vi "Config.vi"(8 "error in (no error)":errorcluster, 9 "Conf. Gral.":T1, 10 "Array Parsed Expression":T3[](array[typedef]), 11 "Variable Data In":T2) -> (0 "error out":errorcluster, 1 "Conf. Gral. Out":T1, 2 "Array Parsed Expression Out":T3[](array[typedef]), 3 "Variable Data Out":T2)   [LabVIEW 2014, in "MathLoop.lvlib"]
doc: "Configura Auxiliares, mediciones, ctes y dimensiones."
uses:
  MathLoop.lvlib
  TypeDefs/ParsedExpression.ctl
  TypeDefs/typeMed.ctl
  TypeDefs/NumericData.ctl
  TypeDefs/Conf. Gral.ctl
panel:
  in  "Configuración General.":bool
  in  "Acept":bool
  in  "Cancelar":bool
  in  "Dimensiones de Patrón":bool
  in  "Constantes de Medición":bool
  in  "Medidas Auxiliares":bool
  in  "Definición de Mediciones M":bool
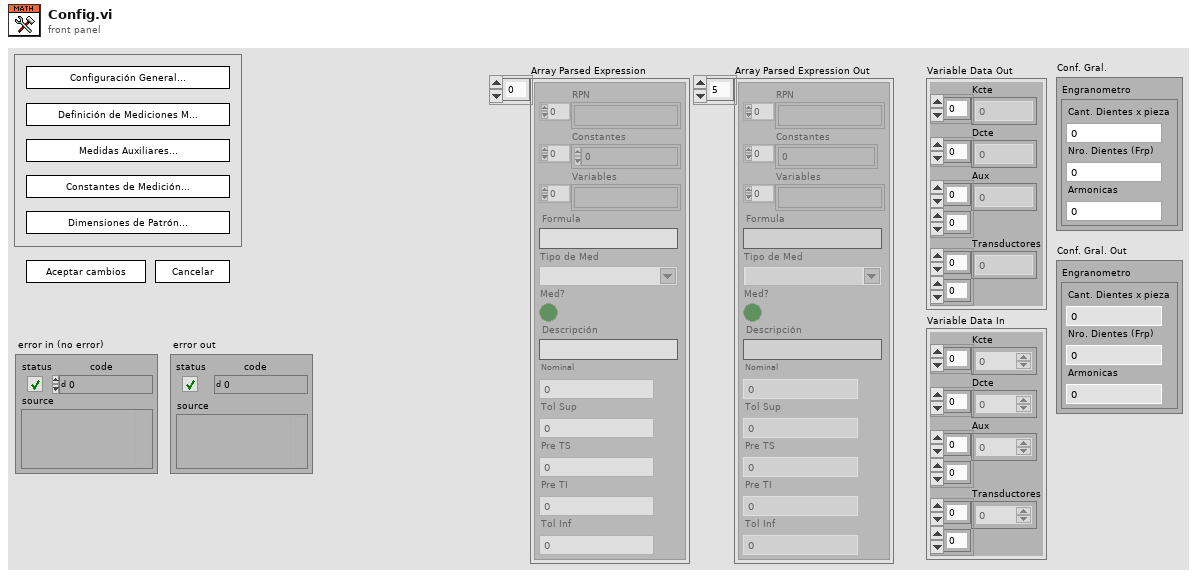
[diagram p1: front panel]
types:
  T1 = typedef "MathLoop.lvlib/Conf. Gral.ctl" = cluster{"Engranometro":cluster{"Cant. Dientes x pieza":i32, "Nro. Dientes (Frp)":i32, "Armonicas":i32}}
  T2 = typedef "MathLoop.lvlib/NumericData.ctl" = cluster{"Kcte":sgl[], "Dcte":sgl[], "Aux":sgl[][], "Transductores":sgl[][]}
  T3 = typedef "MathLoop.lvlib/ParsedExpression.ctl" = cluster{"RPN ":string[], "Constantes":sgl[], "Variables":string[], "Formula":string, "Tipo de Med":T4, "Med?":bool, "Descripción":string, "Nominal":sgl, "Tol Sup":sgl, "Pre TS":sgl, "Pre TI":sgl, "Tol Inf":sgl}
  T4 = typedef "MathLoop.lvlib/typeMed.ctl" = string
  T5 = cluster{"Kcte":sgl[], "Dcte":sgl[], "Aux":sgl[][], "Transductores":sgl[][]}
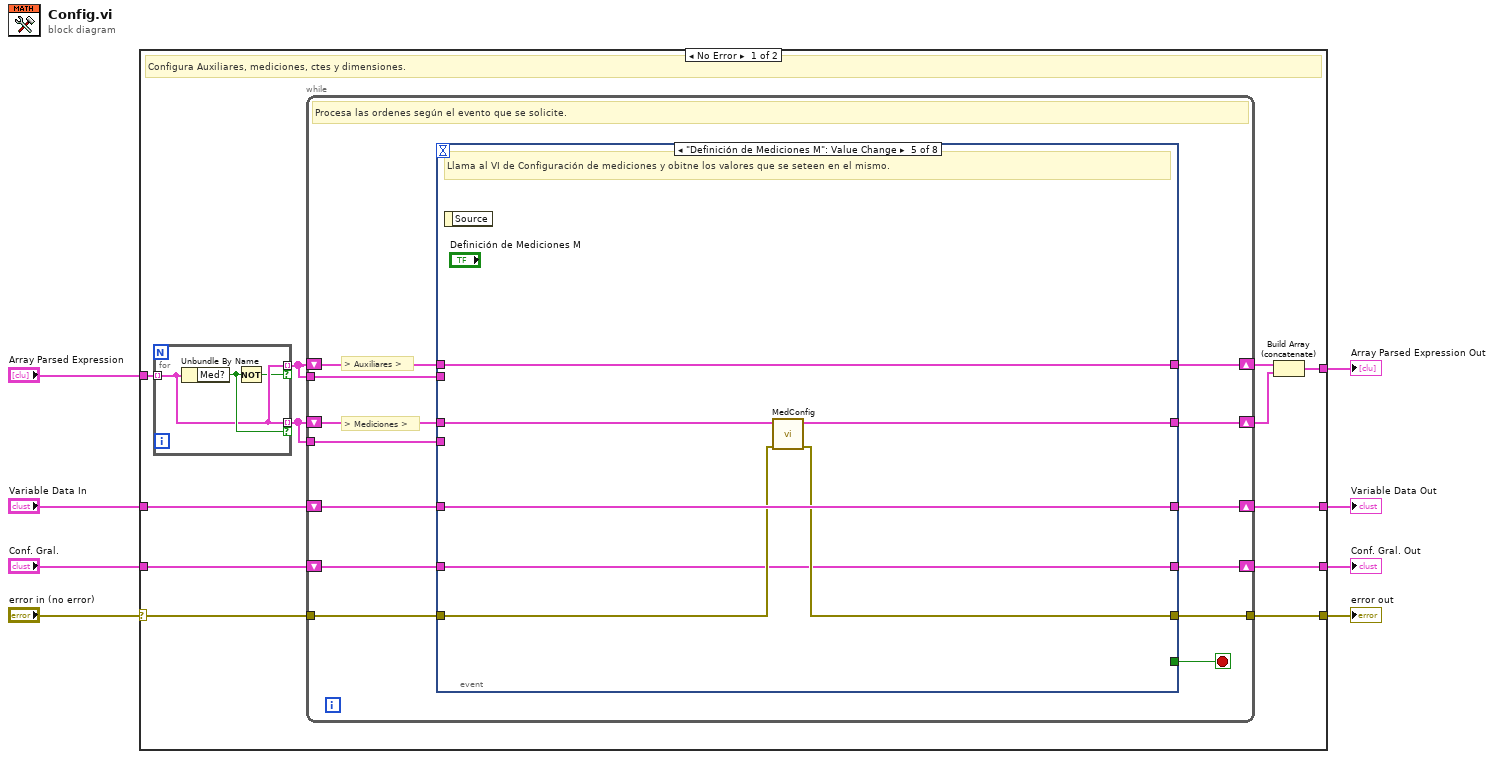
[diagram p0: block diagram]
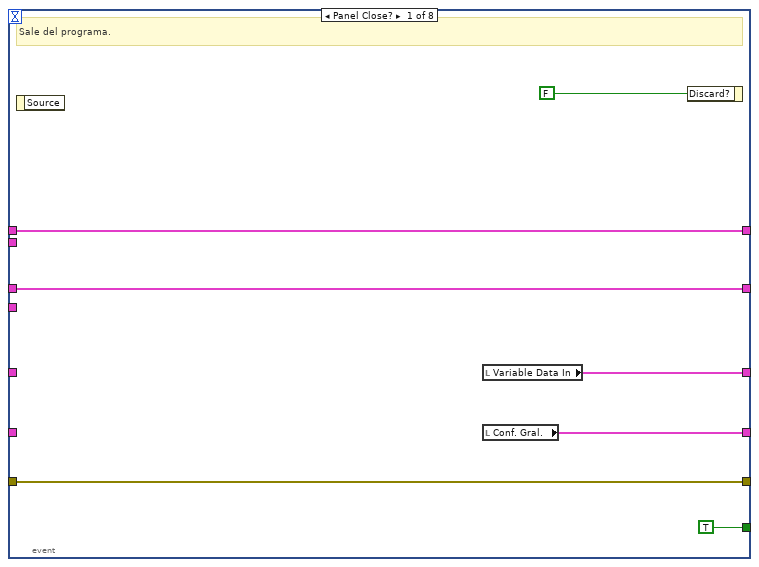
[diagram p2: hidden frame]
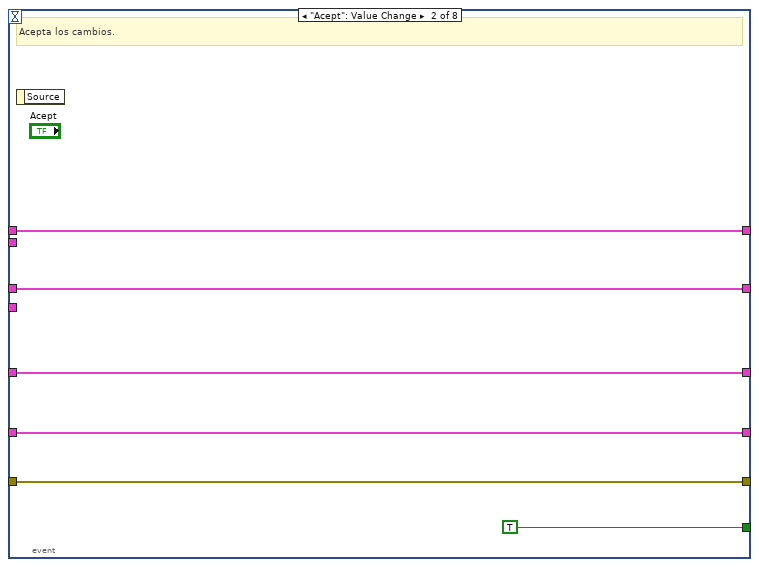
[diagram p3: hidden frame]
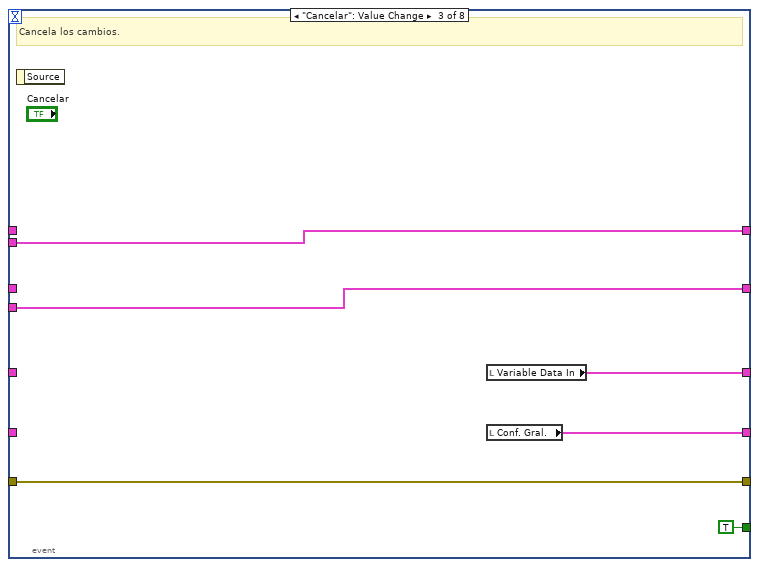
[diagram p4: hidden frame]
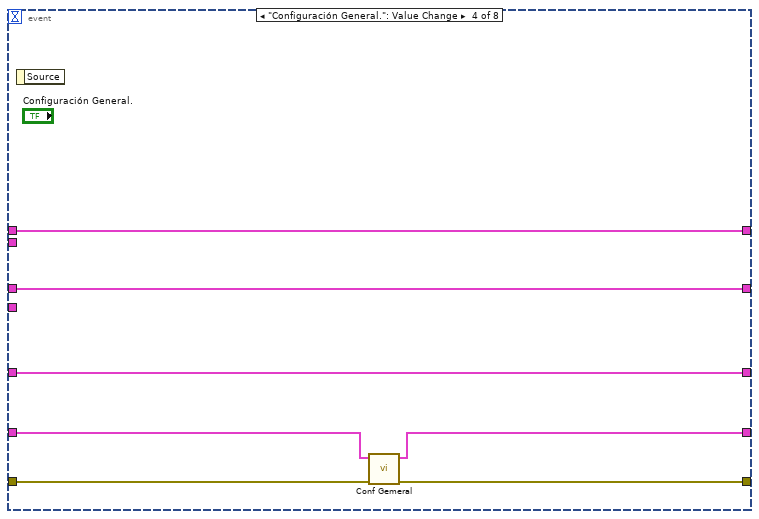
[diagram p5: hidden frame]
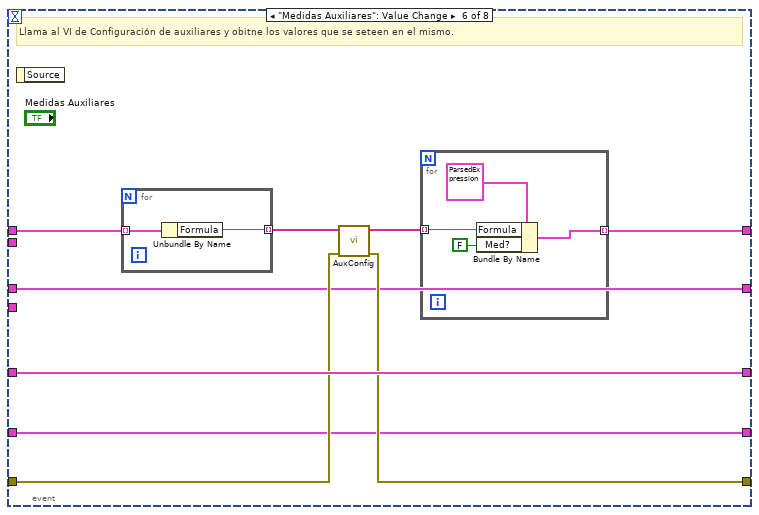
[diagram p6: hidden frame]
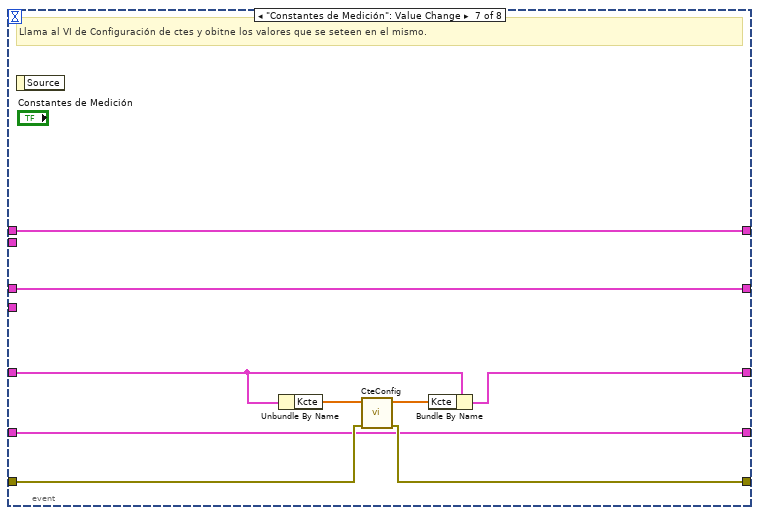
[diagram p7: hidden frame]
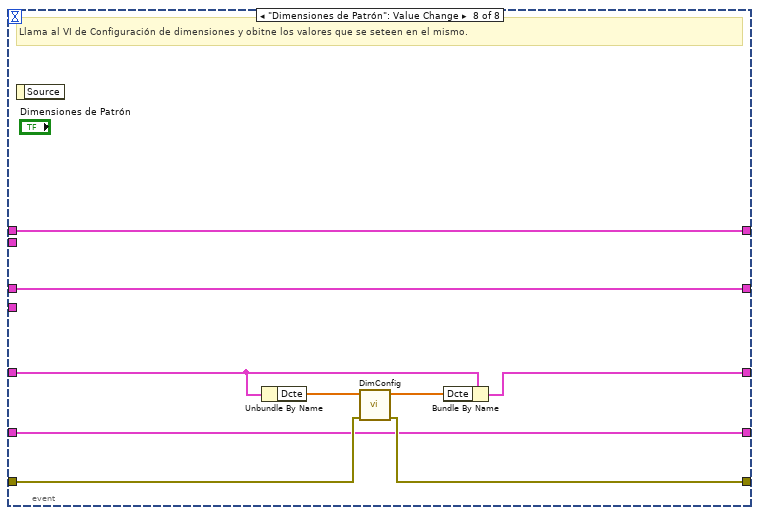
[diagram p8: hidden frame]
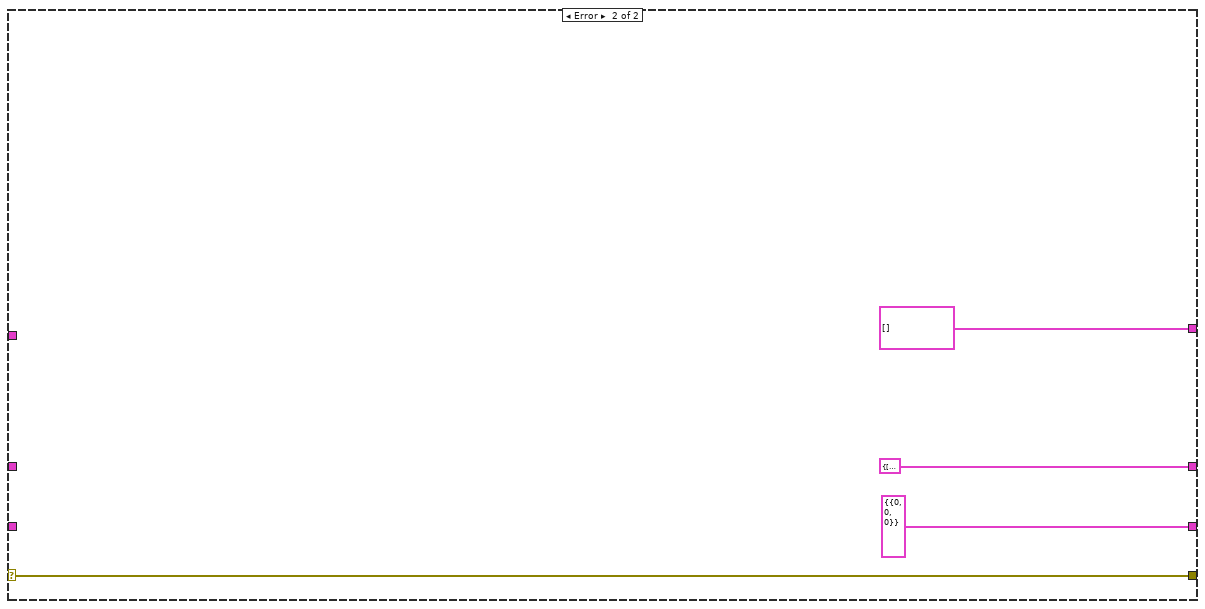
[diagram p9: hidden frame]
diagram:
  n1 = case shown="No Error" "error in (no error)" {
    selector: "error in (no error)" -> [w20 w106]
    tunnel: [w17 w106] -> w7
    tunnel: "Variable Data In" -> [w18 _]
    tunnel: "Array Parsed Expression" -> [w13 _]
    tunnel: [w19 T5 {"Kcte"=[], "Dcte"=[], "Aux"=[], "Transductores"=[]} ("Variable Data")] -> w3
    tunnel: [w14 T3[] [] ("Array Parsed Expression")] -> w5
    tunnel: [w10 T1 {"Engranometro"={"Cant. Dientes x pieza"=0, "Nro. Dientes (Frp)"=0, "Armonicas"=0}} ("Conf. Gral.")] -> w2
    tunnel: "Conf. Gral." -> [w9 _]
    frame No Error {
      # "Configura Auxiliares, mediciones, ctes y dimensiones."
      n2 = for {
        tunnel: w13 -> [w22] mode=indexing
        tunnel: [w22] -> w11 mode=indexing if=w23
        tunnel: [w22] -> w12 mode=indexing if=w21
        n3 = Unbundle By Name(w22) -> ("Med?"=w23:bool)
        n4 = Not(x=w23) -> (.not. x?=w21:bool)
      }
      n5 = while {
        tunnel: w20 -> [w36]
        tunnel: [w32] -> w17
        shift-right: [w33] -> w19
        shift-left: w18 -> [w34]
        shift-right: [w31] -> w16
        shift-left: w12 -> [w30]
        shift-right: [w29] -> w15
        shift-left: w11 -> [w28]
        tunnel: w12 -> [w27]
        tunnel: w11 -> [w26]
        shift-right: [w25] -> w10
        shift-left: w9 -> [w24]
        stop <- w35 stop-if-true
        # "> Mediciones >"
        # "> Auxiliares >"
        # "Procesa las ordenes según el evento que se solicite."
        n6 = event shown="[4] \"Definición de Mediciones M\": Value Change" {
          selector: _ -> [_ _ _ _ _ _ _ _]
          dyn-events: _ -> [_ _ _ _ _ _ _ _]
          timeout: _ -> [_ _ _ _ _ _ _ _]
          tunnel: [w42 w48 w55 w58 w66 w75 w90 w102] -> w32
          tunnel: w36 -> [w42 w48 w55 w59 w67 w76 w91 w101]
          tunnel: [TRUE ("Guardar") TRUE ("Guardar") TRUE ("Guardar") _ _ _ _ _] -> w35
          tunnel: w34 -> [_ w46 _ w62 w69 w78 w93 w100]
          tunnel: [w40 w46 w53 w62 w69 w78 w92 w99] -> w33
          tunnel: [w39 w47 w52 w61 w68 w72 w89 w98] -> w31
          tunnel: w30 -> [w39 w47 _ w61 w68 w71 w89 w98]
          tunnel: [w38 w45 w51 w60 w65 w74 w86 w95] -> w29
          tunnel: w28 -> [w38 w45 _ w60 w64 w74 w86 w95]
          tunnel: w27 -> [_ _ w52 _ _ _ _ _]
          tunnel: w26 -> [_ _ w51 _ _ _ _ _]
          tunnel: [w37 w44 w50 w57 w63 w70 w85 w94] -> w25
          tunnel: w24 -> [_ w44 _ w56 w63 w70 w85 w94]
          event Panel Close? {
            # "Sale del programa."
            n7 = event-data() -> ()  [unwired: 1 in, 1 out]
            n8 = local read "Variable Data In"() -> (w40:T2)
            n9 = local read "Conf. Gral."() -> (w37:T1)
            n10 = event-data("Discard?"=FALSE) -> ()  [unwired: 1 in, 1 out]
          }
          event "Acept": Value Change {
            # "Acepta los cambios."
            n11 = event-data() -> ()  [unwired: 1 in, 1 out]
          }
          event "Cancelar": Value Change {
            # "Cancela los cambios."
            n12 = event-data() -> ()  [unwired: 1 in, 1 out]
            n13 = local read "Variable Data In"() -> (w53:T2)
            n14 = local read "Conf. Gral."() -> (w50:T1)
          }
          event "Configuración General.": Value Change {
            n15 = event-data() -> ()  [unwired: 1 in, 1 out]
            n16 = call "Conf Gemeral.vi"("error in (no error)"=w59, "Conf. Gral."=w56) -> ("error out"=w58:errorcluster, "Conf. Gral. Out"=w57:T1)  [unwired: 8 in]
          }
          event "Definición de Mediciones M": Value Change {
            # "Llama al VI de Configuración de mediciones y obitne los valores que se seteen en el mismo."
            n17 = event-data() -> ()  [unwired: 1 in, 1 out]
            n18 = call "MedConfig.vi"("error in (no error)"=w67, "Array Parsed Expression"=w64) -> ("error out"=w66:errorcluster, "Array Parsed Expression Out"=w65:T3[])  [unwired: 8 in]
          }
          event "Medidas Auxiliares": Value Change {
            # "Llama al VI de Configuración de auxiliares y obitne los valores que se seteen en el mismo."
            n19 = event-data() -> ()  [unwired: 1 in, 1 out]
            n20 = for {
              tunnel: w71 -> [w84] mode=indexing
              tunnel: [w83] -> w77 mode=indexing
              n21 = Unbundle By Name(w84) -> ("Formula"=w83:string)
            }
            n22 = call "AuxConfig.vi"("error in (no error)"=w76, "Aux in"=w77) -> ("error out"=w75:errorcluster, "Aux"=w73:string[])  [unwired: 8 in]
            n23 = for {
              tunnel: w73 -> [w81] mode=indexing
              tunnel: [w80] -> w72 mode=indexing
              n24 = Bundle By Name(cluster=T3 {"RPN "=[], "Constantes"=[], "Variables"=[], "Formula"="", "Tipo de Med"="", "Med?"=FALSE, "Descripción"="", "Nominal"=0.0, "Tol Sup"=0.0, "Pre TS"=0.0, "Pre TI"=0.0, "Tol Inf"=0.0} ("Parsed Expression"), "Formula"=w81, "Med?"=FALSE) -> (w80:T3)
            }
          }
          event "Constantes de Medición": Value Change {
            # "Llama al VI de Configuración de ctes y obitne los valores que se seteen en el mismo."
            n25 = event-data() -> ()  [unwired: 1 in, 1 out]
            n26 = Unbundle By Name(w93) -> ("Kcte"=w87:sgl[])
            n27 = call "CteConfig.vi"("error in (no error)"=w91, "Cte in"=w87) -> ("error out"=w90:errorcluster, "Cte"=w88:sgl[])  [unwired: 8 in]
            n28 = Bundle By Name(cluster=w93, "Kcte"=w88) -> (w92:T2)
          }
          event "Dimensiones de Patrón": Value Change {
            # "Llama al VI de Configuración de dimensiones y obitne los valores que se seteen en el mismo."
            n29 = event-data() -> ()  [unwired: 1 in, 1 out]
            n30 = Unbundle By Name(w100) -> ("Dcte"=w97:sgl[])
            n31 = call "DimConfig.vi"("error in (no error)"=w101, "Dim in"=w97) -> ("error out"=w102:errorcluster, "Dim"=w96:sgl[])  [unwired: 8 in]
            n32 = Bundle By Name(cluster=w100, "Dcte"=w96) -> (w99:T2)
          }
        }
      }
      n33 = Build Array (concatenate)(w16, w15) -> (w14:T3[])
    }
    frame Error {
    }
  }
  "error out" <- w7
  "Array Parsed Expression Out" <- w5
  "Variable Data Out" <- w3
  "Conf. Gral. Out" <- w2
